vi "ReadCampaignXML.vi"() -> (3 "Campaign Data":cluster{})   [LabVIEW 2012]
uses:
  <vilib>/Utility/xml.llb/Read From XML File(string).vi
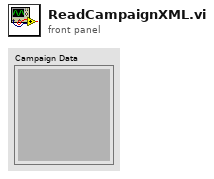
[diagram p1: front panel]
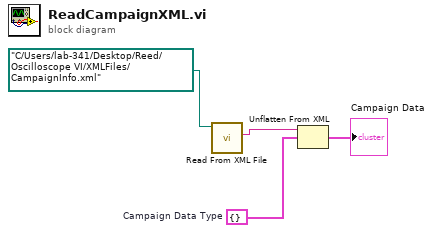
[diagram p0: block diagram]
diagram:
  w1 = cluster{} {}  # Campaign Data Type
  n1 = call-poly <vilib>:"Read From XML File.vi"("XML File Path"=path "C:/Users/lab-341/Desktop/Reed/Oscilloscope VI/XMLFiles/CampaignInfo.xml") -> ("XML Elements"=w3:string)  [unwired: 8 in, 2 out]
  n2 = Unflatten From XML(xml string=w3, type=w1) -> (value=→"Campaign Data":cluster{})  [unwired: 1 in, 1 out]
